vi "MFC Launcher.vi"(9 "Sub Panel":refnum<vi>, 10 "MFC ID":enum16{"Inner Flow", "Outer Flow"}(ring), 11 "Panel Actor In":refnum<class "Main.lvclass">) -> (2 "Nested Actor's Enqueuer":refnum<class "Message Enqueuer.lvclass">, 3 "Panel Actor Out":refnum<class "Main.lvclass">)   [LabVIEW 2018, in "MFC Actor.lvlib" / "MFC.lvclass"]
uses:
  MFC.lvclass
  ADM/ADM/Main.lvclass
  C:/Program Files/National Instruments/LabVIEW 2018/vi.lib/MGI/Panel Manager/Panel Actor/Panel Actor/Panel Actor.lvclass
  <vilib>/ActorFramework/Message Enqueuer/Message Enqueuer.lvclass
  MFC.lvclass/MFC.ctl
  <vilib>/MGI/Panel Manager/Panel/Panel/Subpanel/Subpanel.lvclass
  C:/Program Files/National Instruments/LabVIEW 2018/vi.lib/MGI/Panel Manager/Panel/Panel/Panel.lvclass
  <vilib>/MGI/Panel Manager/Panel/Panel/Subpanel/Subpanel.vi
  <vilib>/MGI/Panel Manager/Panel/Panel.lvlib
  <vilib>/MGI/Panel Manager/Panel Actor/Panel Actor/Panel Actor.lvclass
  <instrlib>/Sierra Instruments Smart-Trak 100 Series/Sierra Instruments Smart-Trak 100 Series.lvlib
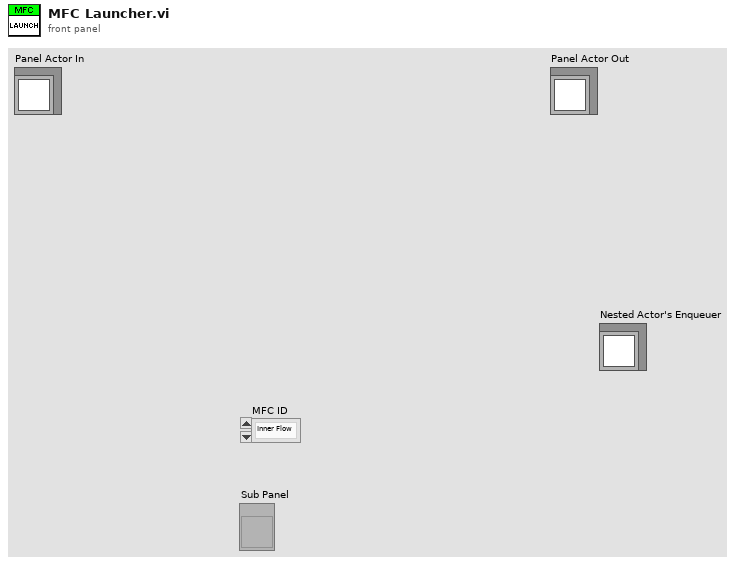
[diagram p1: front panel]
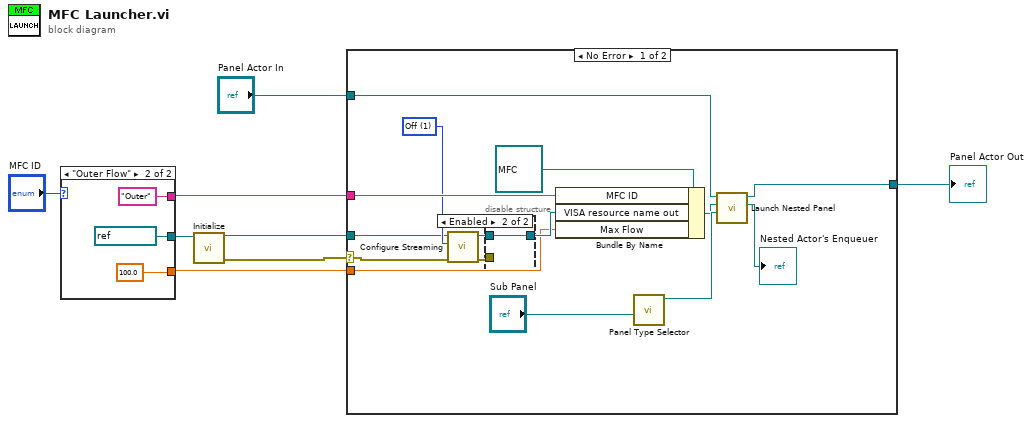
[diagram p0: block diagram]
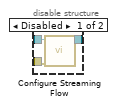
[diagram p2: hidden frame]
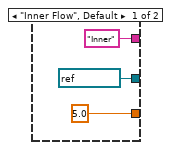
[diagram p4: hidden frame]
diagram:
  n1 = case shown="\"Outer Flow\"" "MFC ID" {
    tunnel: ["Inner" "Outer"] -> w7
    tunnel: [refnum<visa-resource-name> "COM2" ("VISA resource name") refnum<visa-resource-name> "COM1" ("VISA resource name")] -> w5
    tunnel: [5.0 100.0] -> w4
    frame "Inner Flow", Default {
    }
    frame "Outer Flow" {
    }
  }
  n2 = call <instrlib>:"Initialize.vi"("VISA resource name"=w5) -> ("error out"=w1:errorcluster, "VISA resource name out"=w6:refnum<visa-resource-name>)  [unwired: 9 in]
  n3 = case shown="No Error" w1 {
    selector: w1 -> [w15 _]
    tunnel: w7 -> [w25 _]
    tunnel: w6 -> [w20 _]
    tunnel: w4 -> [w18 _]
    tunnel: "Panel Actor In" -> [w17 w34]
    tunnel: [w16 w34] -> w2
    frame No Error {
      w23 = u16 1 items=["On", "Off", "Echo"] ("Streaming Mode (0: On)")
      n4 = call <instrlib>:"Configure Streaming.vi"("error in (no error)"=w15, "Streaming Mode (0: On)"=w23, "VISA resource name"=w20) -> ("error out"=w22:errorcluster, "VISA resource name out"=w21:refnum<visa-resource-name>)  [unwired: 7 in]
      n5 = disable-structure shown="Enabled" {
        disable-tunnel: w22 -> [w32 _]
        disable-tunnel: w21 -> [w31 w33]
        disable-tunnel: [w30 w33] -> w19
        frame Disabled {
          n6 = call <instrlib>:"Configure Streaming Flow.vi"("error in (no error)"=w32, "VISA resource name"=w31) -> ("VISA resource name out"=w30:refnum<visa-resource-name>)  [unwired: 8 in, 1 out]
        }
        frame Enabled {
        }
      }
      n7 = Bundle By Name(cluster=refnum<class "MFC.lvclass"> refnum ("MFC Actor.lvlib:MFC.lvclass"), "MFC ID"=w25, "VISA resource name out"=w19, "Max Flow"=w18) -> (w26:refnum<class "MFC.lvclass">)
      n8 = call-poly <vilib>:"Panel Type Selector.vi"("Sub Panel"="Sub Panel") -> ("Subpanel Out"=w27:refnum<class "Subpanel.lvclass">)  [unwired: 9 in, 1 out]
      n9 = call <vilib>:"Launch Nested Panel.vi"("Panel"=w27, "Nested Panel Actor"=w26, "Panel Actor in"=w17) -> ("Nested Actor's Enqueuer"=→"Nested Actor's Enqueuer":refnum<class "Message Enqueuer.lvclass">, "Panel Actor out"=w16:refnum<class "Main.lvclass">)  [unwired: 5 in, 2 out]
    }
    frame Error {
    }
  }
  "Panel Actor Out" <- w2
